vi "Read Analog Input.vi"(4 "MASTER in":T1 {"Image data"."Color Palette" items=["Grayscale U8", "False Color", "Overexposed"]; "Image data"."Exposure time [us]" format="%#_10g"; "Queue"."Initial time [s]" format="%_19f"; "Queue"."Raw data [V]\n(all samples)" format="%0.2f"; "Queue"."Timestamp [s]" format="%_19f"}) -> (1 "MASTER out":T1 {"Image data"."Color Palette" items=["Grayscale U8", "False Color", "Overexposed"]; "Image data"."Exposure time [us]" format="%#_10g"; "Queue"."Initial time [s]" format="%_19f"; "Queue"."Raw data [V]\n(all samples)" format="%0.2f"; "Queue"."Timestamp [s]" format="%_19f"})   [LabVIEW 2020]
uses:
  MASTER.ctl
  Constants.ctl
  QBundle.ctl
  Queue.ctl
  Image data.ctl
  <vilib>/userdefined/High Color/IMAQdx.ctl
  <vilib>/vision/Image Controls.llb/IMAQ Image.ctl
  Image QBundle.ctl
  <vilib>/DAQmx/read.llb/DAQmx Read (Analog 2D DBL NChan NSamp).vi
  <vilib>/DAQmx/miscellaneous.llb/DAQmx Fill In Error Info.vi
  <resource>/objmgr/daqmx.rc
panel:
  out "AvailSampPerChan":u32
  # "Description:\nUses DAQmx read function to read NChan and NSamp for analog input DAQmx task. Averages NSamp for each channel."
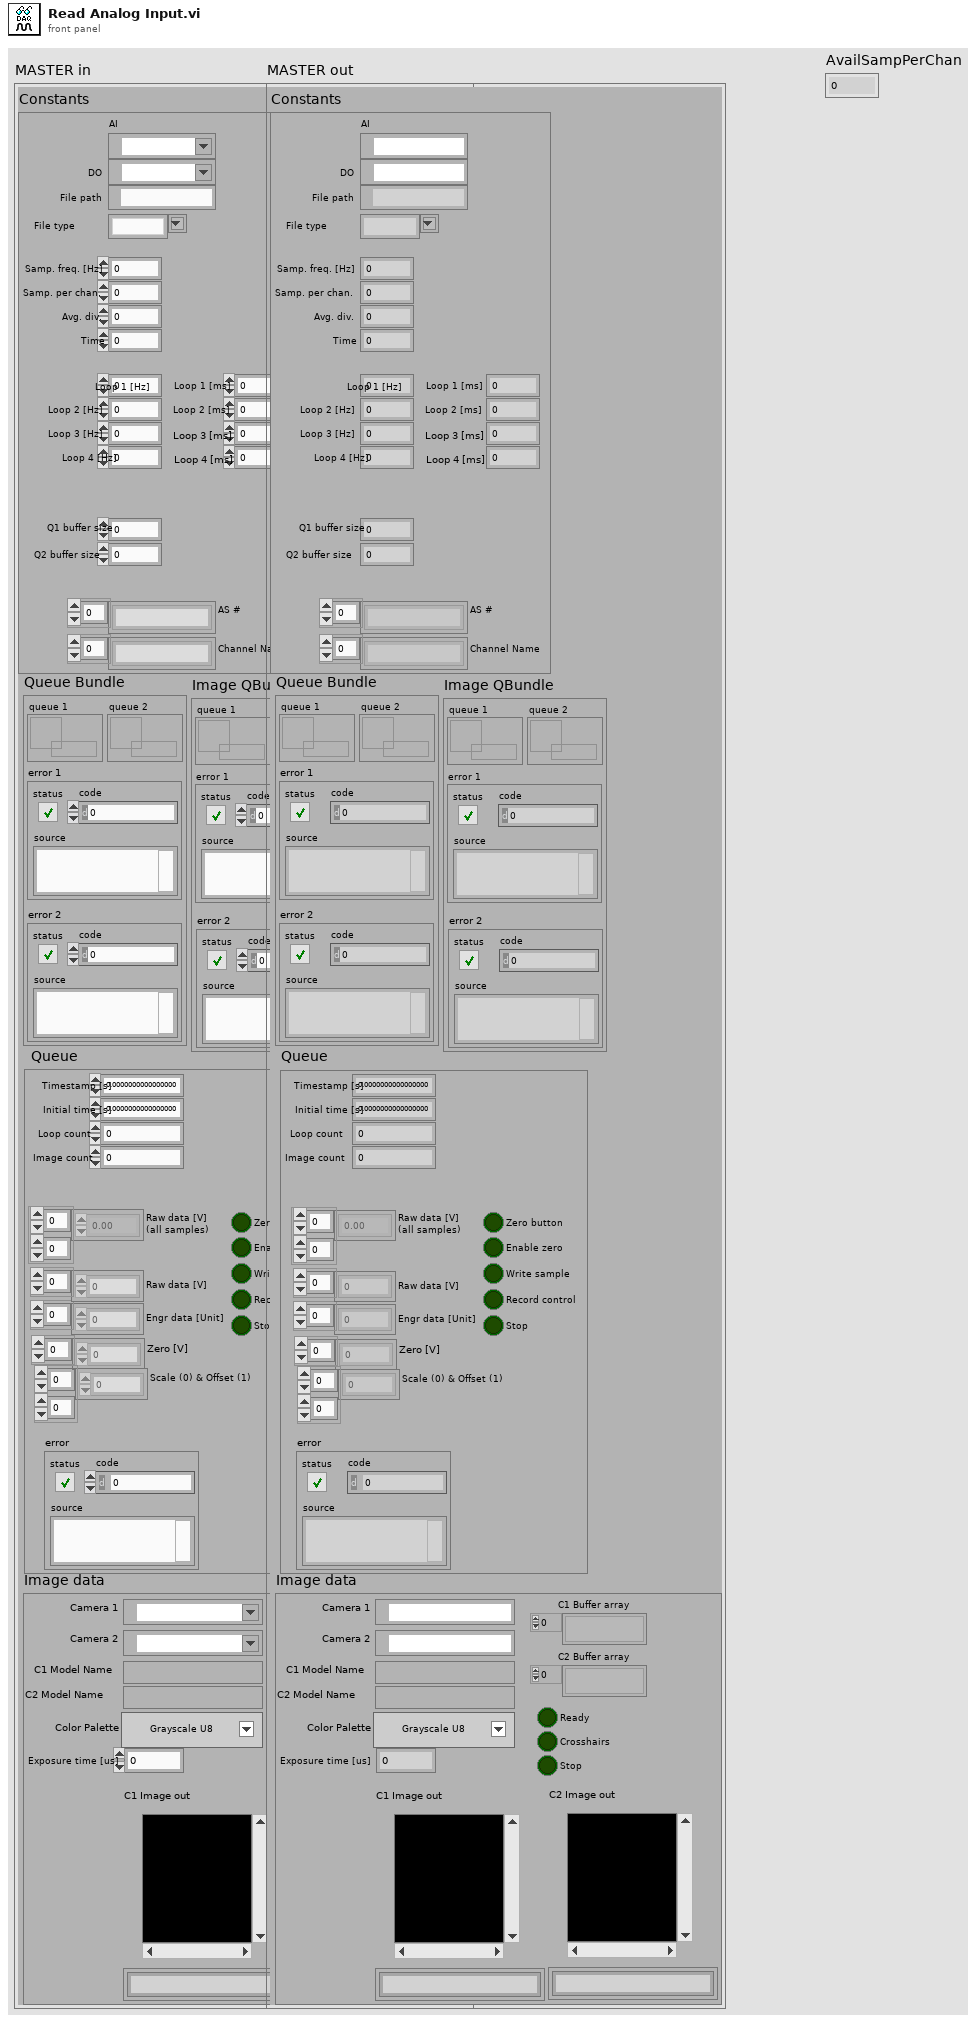
[diagram p1: front panel]
types:
  T1 = typedef "MASTER.ctl" = cluster{"Constants":T2, "Queue Bundle":T3, "Queue":T4, "Image data":T5, "Image QBundle ":T8}
  T2 = typedef "Constants.ctl" = cluster{"Time":u16, "Samp. freq. [Hz]":dbl, "Samp. per chan.":i32, "Avg. div.":i32, "File path":path, "AI":refnum<k21>, "Loop 1 [Hz]":dbl, "Loop 2 [Hz]":dbl, "Loop 3 [Hz]":dbl, "Loop 1 [ms]":dbl, "Loop 2 [ms]":dbl, "Loop 3 [ms]":dbl, "Q1 buffer size":i32, "Q2 buffer size":i32, "File type":string, "Loop 4 [Hz]":dbl, "Loop 4 [ms]":dbl, "Channel Name":string[], "AS #":string[], "DO":refnum<k21>}
  T3 = typedef "QBundle.ctl" = cluster{"queue 1":refnum<queue>, "error 1":errorcluster, "queue 2":refnum<queue>, "error 2":errorcluster}
  T4 = typedef "Queue.ctl" = cluster{"Enable zero":bool, "Engr data [Unit]":dbl[], "Zero button":bool, "Zero [V]":dbl[], "Timestamp [s]":dbl, "Write sample":bool, "Record control":bool, "Stop":bool, "error":errorcluster, "Raw data [V]\n(all samples)":dbl[][], "Raw data [V]":dbl[], "Loop count":i64, "Initial time [s]":dbl, "Scale (0) & Offset (1)":dbl[][], "Image count":dbl}
  T5 = typedef "Image data.ctl" = cluster{"Camera 1":T6, "Camera 2":T6, "C1 Image out ":T7, "C2 Image out":T7, "C1 Model Name":string, "C2 Model Name":string, "Exposure time [us]":dbl, "Color Palette":u16, "C1 Buffer array":T7[], "Ready":bool, "C2 Buffer array":T7[], "Crosshairs":bool, "Stop":bool}
  T6 = typedef "IMAQdx.ctl" = refnum<k21>
  T7 = typedef "IMAQ Image.ctl" = refnum<image>
  T8 = typedef "Image QBundle.ctl" = cluster{"queue 1":refnum<queue>, "error 1":errorcluster, "queue 2":refnum<queue>, "error 2":errorcluster}
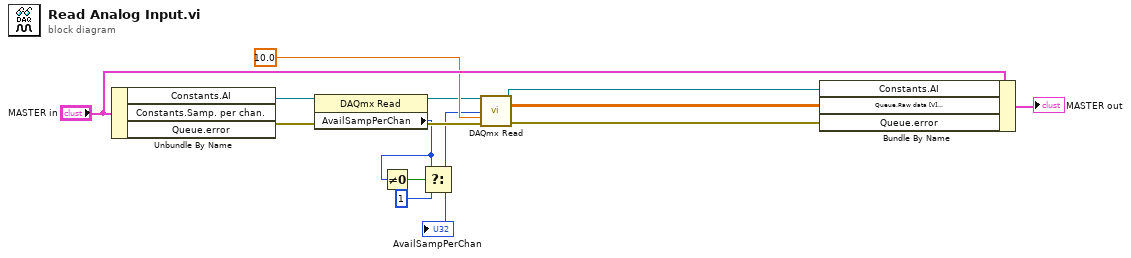
[diagram p0: block diagram]
diagram:
  n1 = Unbundle By Name("MASTER in") -> ("Constants.AI"=w10:refnum<k21>, "Queue.error"=w13:errorcluster)  [unwired: 1 out]
  n2 = property class="DAQmx Read"(reference=w10) -> (reference out=w5:refnum<k21>, "AvailSampPerChan"=w3:u32)  [unwired: 1 in, 1 out]
  n3 = Not Equal To 0?(x=w3) -> (x != 0?=w4:bool)
  n4 = Select(t=w3, s=w4, f=u32 1) -> (s? t:f=w1:u32)
  "AvailSampPerChan" <- w1
  n5 = call-poly <vilib>:"DAQmx Read.vi"("task/channels in"=w5, "number of samples per channel"=w1, "timeout"=10.0, "error in"=w13) -> ("task out"=w12:refnum<k21>, "data"=w7:dbl[][], "error out"=w8:errorcluster)  [unwired: 9 in]
  n6 = Bundle By Name(cluster="MASTER in", "Constants.AI"=w12, "Queue.Raw data [V]\n(all samples)"=w7, "Queue.error"=w8) -> (→"MASTER out":T1)
